vi "tiffWriteImaqToTiff.vi"(6 "ImageDescription":string, 7 "Compress?":bool=TRUE, 9 "Multipage":cluster{"Page":i32, "TotalPages":i32}, 10 "ImaqIn":T1, 11 "TiffIn":refnum<k24>) -> (2 "ImaqOut":T1, 3 "TiffOut":refnum<k24>)   [LabVIEW 2022 SP3, in "LVTiffWriter.lvlib"]
doc: "This VI writes on page/directory to the tiff file opened with tiffOpenForWrite.\n\nWire the current page index and total number of pages if you want to do multitiff."
uses:
  LVTiffWriter.lvlib
  <vilib>/vision/Image Controls.llb/IMAQ Image.ctl
  C:/Nuget/BitMiracle.LibTiff.NET.2.4.649/lib/net40/BitMiracle.LibTiff.NET.dll
  Nuget/BitMiracle.LibTiff.NET.2.4.649/lib/net40/BitMiracle.LibTiff.NET.dll
panel:
  out "BytesPerStrip":i32
  in  "BytesPerStrip\nWanted":i32=16384
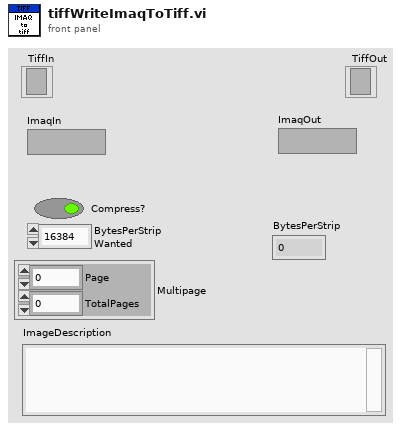
[diagram p1: front panel]
types:
  T1 = typedef "IMAQ Image.ctl" = refnum<image>
  T2 = cluster{"ImageWidth":i32, "ImageLength":i32, "RowsPerStrip":i32}
  T3 = typedef "Image Type" = u32
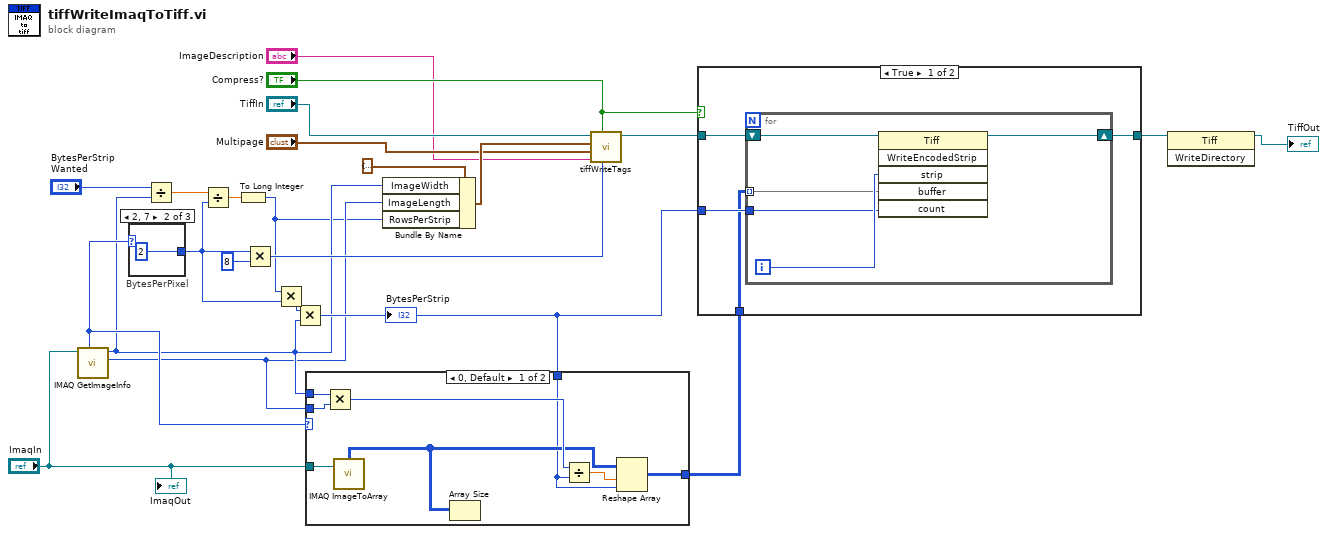
[diagram p0: block diagram]
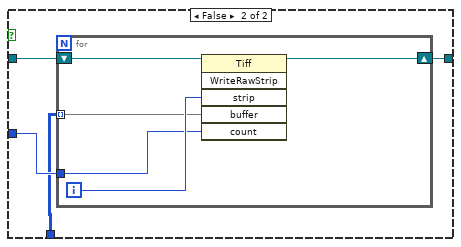
[diagram p2: hidden frame]
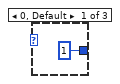
[diagram p3: hidden frame]
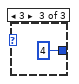
[diagram p4: hidden frame]
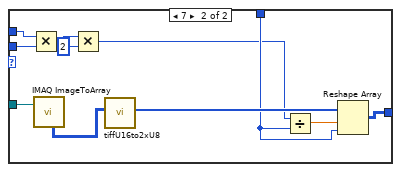
[diagram p5: hidden frame]
diagram:
  n1 = call "IMAQ GetImageInfo"("Image"="ImaqIn") -> ("Y Resolution"=w8:i32, "X Resolution"=w9:i32, "Image Type"=w20:T3)  [unwired: 3 in, 5 out]
  n2 = case "BytesPerPixel" shown="2, 7" w20 {
    tunnel: [1 2 4] -> w17
    frame 0, Default {
    }
    frame 2, 7 {
    }
    frame 3 {
    }
  }
  n3 = Divide(x="BytesPerStrip\nWanted", y=w9) -> (x/y=w13:dbl)
  n4 = Divide(x=w13, y=w17) -> (x/y=w14:dbl)
  n5 = To Long Integer(number=w14) -> (32bit integer=w7:i32)
  n6 = Multiply(x=w17, y=8) -> (x*y=w16:i32)
  n7 = Multiply(x=w7, y=w17) -> (x*y=w18:i32)
  n8 = Multiply(x=w18, y=w9) -> (x*y=w22:i32)
  "BytesPerStrip" <- w22
  n9 = case shown="0, Default" w20 {
    tunnel: w8 -> [w32 w41]
    tunnel: w9 -> [w33 w42]
    tunnel: "ImaqIn" -> [w34 w45]
    tunnel: w22 -> [w27 w38]
    tunnel: [w30 w44] -> w23
    frame 0, Default {
      n10 = Multiply(x=w33, y=w32) -> (x*y=w31:i32)
      n11 = call "IMAQ ImageToArray"("Image"=w34) -> ("Image Pixels (U8)"=w29:u8[][])  [unwired: 3 in, 4 out]
      n12 = Array Size(array=w29) -> ()  [unwired: 1 out]
      n13 = Divide(x=w31, y=w27) -> (x/y=w28:dbl)
      n14 = Reshape Array(w29, w28, w27) -> (w30:u8[][])
    }
    frame 7 {
      n15 = Multiply(x=w42, y=w41) -> (x*y=w37:i32)
      n16 = call "IMAQ ImageToArray"("Image"=w45) -> ("Image Pixels (U16)"=w40:u16[][])  [unwired: 3 in, 4 out]
      n17 = Multiply(x=w37, y=2) -> (x*y=w36:i32)
      n18 = call "tiffU16to2xU8.vi"("U16"=w40) -> ("Bytes"=w43:u8[])  [unwired: 10 in]
      n19 = Divide(x=w36, y=w38) -> (x/y=w39:dbl)
      n20 = Reshape Array(w43, w39, w38) -> (w44:u8[][])
    }
  }
  n21 = Bundle By Name(cluster=T2 {"ImageWidth"=0, "ImageLength"=0, "RowsPerStrip"=0} ("Dimensions"), "ImageWidth"=w9, "ImageLength"=w8, "RowsPerStrip"=w7) -> (w5:T2)
  n22 = call "tiffWriteTags.vi"("BitsPerSample"=w16, "Compress?"="Compress?", "ImageDescription"="ImageDescription", "Multipage"="Multipage", "Dimensions"=w5, "BitMiracle.LibTiff.Classic.Tiff"="TiffIn") -> ("BitMiracle.LibTiff.Classic.Tiff"=w11:refnum<k24>)  [unwired: 5 in]
  n23 = case shown="True" "Compress?" {
    tunnel: w11 -> [w49 w58]
    tunnel: [w48 w57] -> w3
    tunnel: w22 -> [w47 w56]
    tunnel: w23 -> [w46 w55]
    frame True {
      n24 = for {
        shift-right: [w53] -> w48
        shift-left: w49 -> [w54]
        tunnel: w46 -> [w50] mode=indexing
        tunnel: w47 -> [w51]
        i -> [w52]
        n25 = invoke class="Tiff" method="WriteEncodedStrip"(reference=w54, "strip"=w52, "buffer"=w50, "count"=w51) -> (reference out=w53:refnum<k24>)  [unwired: 2 in, 5 out]
      }
    }
    frame False {
      n26 = for {
        shift-right: [w62] -> w57
        shift-left: w58 -> [w63]
        tunnel: w56 -> [w60]
        tunnel: w55 -> [w59] mode=indexing
        i -> [w61]
        n27 = invoke class="Tiff" method="WriteRawStrip"(reference=w63, "strip"=w61, "buffer"=w59, "count"=w60) -> (reference out=w62:refnum<k24>)  [unwired: 2 in, 5 out]
      }
    }
  }
  n28 = invoke class="Tiff" method="WriteDirectory"(reference=w3) -> (reference out=→"TiffOut":refnum<k24>)  [unwired: 2 in, 2 out]
  "ImaqOut" <- "ImaqIn"
